vi "_PC_Pub_Conv_ColorHexNum.vi"(3 "HexStringIn":string) -> (0 "ErrorBool":bool, 1 "HexNumOut":u32)   [LabVIEW 2018]
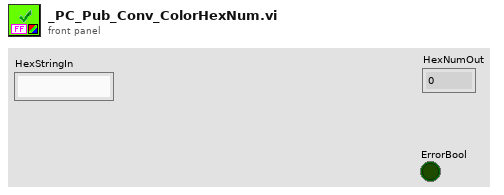
[diagram p1: front panel]
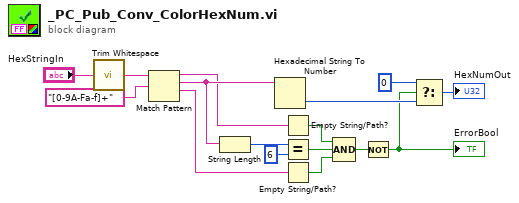
[diagram p0: block diagram]
diagram:
  n1 = call <vilib>:"Trim Whitespace.vi"("string"="HexStringIn") -> ("trimmed string"=w14:string)  [unwired: 1 in]
  n2 = Match Pattern(string=w14, regular expression="[0-9A-Fa-f]+") -> (before substring=w10:string, match substring=w11:string, after substring=w9:string)  [unwired: 1 in, 1 out]
  n3 = String Length(string=w11) -> (length=w13:i32)
  n4 = Hexadecimal String To Number(string=w11) -> (number=w4:u32)  [unwired: 2 in, 1 out]
  n5 = Empty String/Path?(string/path=w10) -> (empty?=w8:bool)
  n6 = Equal?(x=w13, y=6) -> (x = y?=w7:bool)
  n7 = Empty String/Path?(string/path=w9) -> (empty?=w6:bool)
  n8 = Compound Arithmetic op=AND(w8, w7, w6) -> (w5:bool)
  n9 = Not(x=w5) -> (.not. x?=w3:bool)
  "ErrorBool" <- w3
  n10 = Select(t=u32 0, s=w3, f=w4) -> (s? t:f=→"HexNumOut":u32)
